vi "solar_app Screenshot.vi"(8 "error in (no error)":errorcluster, 9 "Additional Info":string[](array[string]), 10 "VI Refnums":refnum<vi>[](array[refnum]), 11 "LogsDir":path) -> (0 "error out":errorcluster, 2 "Filenames":string[](array[string]), 3 "ExportDir":path)   [LabVIEW 2018]
doc: "This exports the VI front panel screenshots (*.png) to the Logs folder"
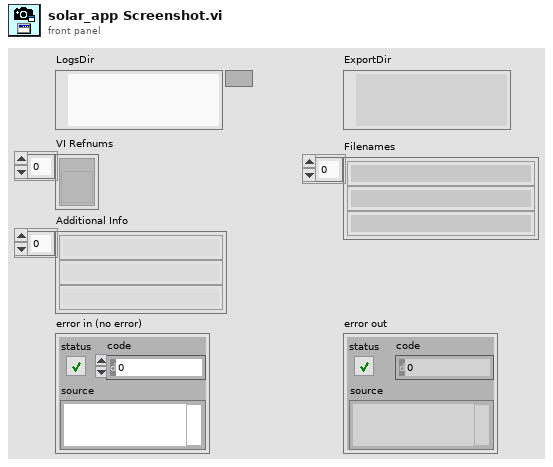
[diagram p1: front panel]
types:
  T1 = cluster{"horizontal":enum16{"left", "center", "right"}, "vertical":enum16{"top", "center", "bottom"}}
  T2 = typedef "imagedata.ctl" = cluster{"image type":i32, "image depth":i32, "image":u8[], "mask":u8[], "colors":u32[], "Rectangle":cluster{"left":i16, "top":i16, "right":i16, "bottom":i16}}
  T3 = cluster{"left":i16, "top":i16, "right":i16, "bottom":i16}
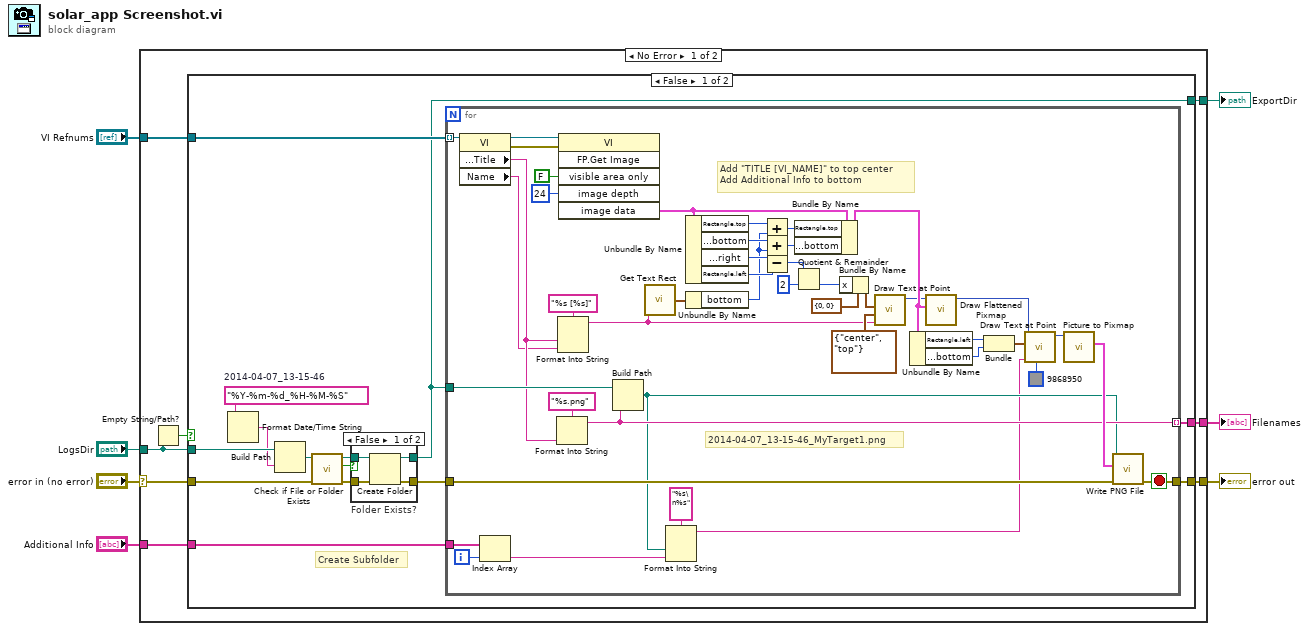
[diagram p0: block diagram]
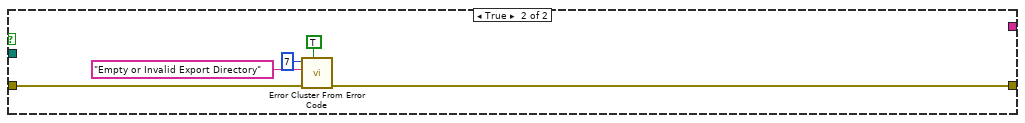
[diagram p3: hidden frame]
diagram:
  n1 = case shown="No Error" "error in (no error)" {
    selector: "error in (no error)" -> [w11 w85]
    tunnel: "VI Refnums" -> [w15 _]
    tunnel: [w14 w85] -> w5
    tunnel: "LogsDir" -> [w10 _]
    tunnel: [w13 _] -> w3
    tunnel: [w12 _] -> w2
    tunnel: "Additional Info" -> [w8 _]
    frame No Error {
      n2 = Empty String/Path?(string/path=w10) -> (empty?=w9:bool)
      n3 = case shown="False" w9 {
        tunnel: w15 -> [w29 _]
        tunnel: [w28 w80] -> w14
        tunnel: [w22 _] -> w13
        tunnel: [w21 _] -> w12
        tunnel: w11 -> [w20 w84]
        tunnel: w10 -> [w19 _]
        tunnel: w8 -> [w18 _]
        frame False {
          w17 = "%Y-%m-%d_%H-%M-%S"  # 2014-04-07_13-15-46
          # "Create Subfolder"
          n4 = Format Date/Time String(time format string (%c)=w17) -> (date/time string=w16:string)  [unwired: 2 in]
          n5 = Build Path(base path=w19, name or relative path=w16) -> (appended path=w23:path)
          n6 = call <vilib>:"Check if File or Folder Exists.vi"("error in (no error)"=w20, "path"=w23) -> ("error out"=w27:errorcluster, "file or folder exists?"=w24:bool, "dup path"=w25:path)  [unwired: 7 in]
          n7 = case "Folder Exists?" shown="False" w24 {
            tunnel: w27 -> [w33 w35]
            tunnel: [w32 w35] -> w26
            tunnel: w25 -> [w31 w34]
            tunnel: [w30 w34] -> w22
            frame False {
              n8 = Create Folder(path (use dialog)=w31, error in=w33) -> (created path=w30:path, error out=w32:errorcluster)  [unwired: 1 in, 1 out]
            }
            frame True {
            }
          }
          n9 = for {
            tunnel: w22 -> [w76]
            tunnel: w26 -> [w75]
            tunnel: [w74] -> w28
            tunnel: w29 -> [w73] mode=indexing
            tunnel: [w66] -> w21 mode=indexing
            tunnel: w18 -> [w68]
            i -> [w67]
            stop <- w74 stop-if-true
            # "Add \"TITLE [VI_NAME]\" to top center\nAdd Additional Info to bottom"
            # "2014-04-07_13-15-46_MyTarget1.png"
            n10 = property class="VI"(reference=w73) -> (reference out=w72:refnum<vi>, error out=w71:errorcluster, "Front Panel.Title"=w55:string, "Name"=w54:string)  [unwired: 1 in]
            n11 = Index Array(array=w68, index=w67) -> (element=w60:string)
            n12 = Format Into String(format string="%s.png", w55) -> (resulting string=w66:string)  [unwired: 2 in, 1 out]
            n13 = Format Into String(format string="%s [%s]", w55, w54) -> (resulting string=w42:string)  [unwired: 2 in, 1 out]
            n14 = invoke class="VI" method="FP.Get Image"(reference=w72, error in=w71, "visible area only"=FALSE ("Visible Area Only"), "image depth"=24 ("Image Depth")) -> ("image data"=w52:T2)  [unwired: 2 in, 5 out]
            n15 = Build Path(base path=w76, name or relative path=w66) -> (appended path=w58:path)
            n16 = call <vilib>:"Get Text Rect.vi"("text"=w42) -> ("rect"=w53:T3)  [unwired: 8 in]
            n17 = Format Into String(format string="%s\n%s", w58, w60) -> (resulting string=w57:string)  [unwired: 2 in, 1 out]
            n18 = Unbundle By Name(w52) -> ("Rectangle.top"=w49:i16, "Rectangle.bottom"=w50:i16, "Rectangle.right"=w46:i16, "Rectangle.left"=w45:i16)
            n19 = Unbundle By Name(w53) -> ("bottom"=w44:i16)
            n20 = Add(x=w49, y=w44) -> (x+y=w48:i16)
            n21 = Add(x=w50, y=w44) -> (x+y=w47:i16)
            n22 = Subtract(x=w46, y=w45) -> (x-y=w40:i16)
            n23 = Quotient & Remainder(x=w40, y=i16 2) -> (floor(x/y)=w36:i16)  [unwired: 1 out]
            n24 = Bundle By Name(cluster=w52, "Rectangle.top"=w48, "Rectangle.bottom"=w47) -> (w51:T2)
            n25 = Bundle By Name(cluster=cluster{"x":i16, "y":i16} {"x"=0, "y"=0} ("origin"), "x"=w36) -> (w37:cluster{"x":i16, "y":i16})
            n26 = call <vilib>:"Draw Text at Point.vi"("text"=w42, "alignment(left, top)"=T1 {"horizontal"=enum."center", "vertical"=enum."top"}, "origin"=w37) -> ("new picture"=w41:picture)  [unwired: 7 in, 1 out]
            n27 = Unbundle By Name(w51) -> ("Rectangle.left"=w63:i16, "Rectangle.bottom"=w62:i16)
            n28 = call <vilib>:"Draw Flattened Pixmap.vi"("image data"=w51, "picture"=w41) -> ("new picture"=w65:picture)  [unwired: 7 in]
            n29 = Bundle("left"=w63, "bottom"=w62) -> (w61:cluster{"left":i16, "bottom":i16})  [unwired: 1 in]
            n30 = call <vilib>:"Draw Text at Point.vi"("text color(black)"=u32 9868950, "text"=w57, "origin"=w61, "picture"=w65) -> ("new picture"=w64:picture)  [unwired: 6 in, 1 out]
            n31 = call <vilib>:"Picture to Pixmap.vi"("picture"=w64) -> ("image data"=w69:T2)  [unwired: 9 in, 1 out]
            n32 = call <vilib>:"Write PNG File.vi"("error in (no error)"=w75, "image data"=w69, "path to PNG file"=w58) -> ("error out"=w74:errorcluster)  [unwired: 7 in, 1 out]
          }
        }
        frame True {
          n33 = call <vilib>:"Error Cluster From Error Code.vi"("show call chain? (False)"=TRUE, "error in (no error)"=w84, "error message (\"\")"="Empty or Invalid Export Directory" ("error message (\"\")"), "error code (0)"=7) -> ("error out"=w80:errorcluster)  [unwired: 5 in]
        }
      }
    }
    frame Error {
    }
  }
  "error out" <- w5
  "ExportDir" <- w3
  "Filenames" <- w2
